vi "Collect Auto V.3.0.vi"() -> (3 "Stop?":bool)   [LabVIEW 2017]
uses:
  2018 Robot Project V.1.0/Robot Global Data.vi
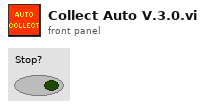
[diagram p1: front panel]
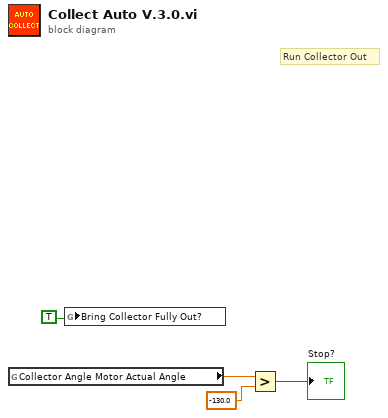
[diagram p0: block diagram]
diagram:
  # "Run Collector Out"
  n1 = global read "Robot Global Data.vi" "Collector Angle Motor Actual Angle"() -> (w3:dbl)
  n2 = global write "Robot Global Data.vi" "Bring Collector Fully Out?"(TRUE) -> ()
  n3 = Greater?(x=w3, y=-130.0) -> (0:→"Stop?":bool)
